vi "test_abs_mixing.vi"() -> ()   [LabVIEW 2017]
doc: "Minimal example that demonstrates functions implemented in the SorpPropLib for absorption working pairs based on the mixing approach."
panel:
  out "Mole fraction of second component":cluster{dbl[], dbl[]}[](graph)=[{[1000.0, 1001.0, 1002.0, 1003.0, 1004.0, 1005.0, 1006.0, 1007.0, 1008.0, 1009.0], [7.283559365756087e-05, 7.276280999979345e-05, 7.26901716201489e-05, 7.261767808386388e-05, 7.254532895861754e-05, 7.247312381253312e-05, 7.24010622172866e-05, 7.232914374399879e-05, 7.225736796756532e-05, 7.218573446365895e-05]}]
  out "Mole fraction of first component":cluster{dbl[], dbl[]}[](graph)=[{[1000.0, 1001.0, 1002.0, 1003.0, 1004.0, 1005.0, 1006.0, 1007.0, 1008.0, 1009.0], [0.9999271644063424, 0.9999272371900002, 0.9999273098283799, 0.9999273823219161, 0.9999274546710414, 0.9999275268761875, 0.9999275989377827, 0.999927670856256, 0.9999277426320324, 0.9999278142655363]}]
  out "Der. of pressure wrt. liquid mole fraction":cluster{dbl[], dbl[]}[](graph)=[{[1000.0, 1001.0, 1002.0, 1003.0, 1004.0, 1005.0, 1006.0, 1007.0, 1008.0, 1009.0], [401367.58805715543, 401367.0721974449, 401385.10792075976, 401372.6104574289, 401380.4616818106, 401371.28151513933, 401381.7575241774, 401382.0286104419, 401375.35766007204, 401370.0730695291]}]
  out "Der. of pressure wrt. temperature":cluster{dbl[], dbl[]}[](graph)=[{[1000.0, 1001.0, 1002.0, 1003.0, 1004.0, 1005.0, 1006.0, 1007.0, 1008.0, 1009.0], [25.245659760457784, 25.27229398367581, 25.296958770582023, 25.321660064605567, 25.347597220388707, 25.374199005341325, 25.39747936339154, 25.424986820326012, 25.4496207963939, 25.4734746010854]}]
  out "Temperature":cluster{dbl[], dbl[]}[](graph)=[{[1000.0, 1001.0, 1002.0, 1003.0, 1004.0, 1005.0, 1006.0, 1007.0, 1008.0, 1009.0], [nan, nan, nan, nan, nan, nan, nan, nan, nan, nan]}]
  out "Pressure":cluster{dbl[], dbl[]}[](graph)=[{[1000.0, 1001.0, 1002.0, 1003.0, 1004.0, 1005.0, 1006.0, 1007.0, 1008.0, 1009.0], [999.9996844004786, 1000.9996848022826, 1001.9996851320313, 1002.9996861115469, 1003.9996864578828, 1004.9996867189573, 1005.9996873328884, 1006.9996881341087, 1007.9996883623128, 1008.9996887136538]}]
  out "Liquid mole fraction":cluster{dbl[], dbl[]}[](graph)=[{[1000.0, 1001.0, 1002.0, 1003.0, 1004.0, 1005.0, 1006.0, 1007.0, 1008.0, 1009.0], [0.0024860925016939863, 0.0024885839313615603, 0.0024910753610397503, 0.002493566790576794, 0.0024960582188671056, 0.002498549646644934, 0.0025010410748412923, 0.0025035325023132905, 0.002506023929378515, 0.002508515355425353]}]
  in  "WorkingPair (Input)":T1={"no_iso"=1, "no_p_sat"=1, "path_db"="D:\\Driesel\\SorpLibLocal\\labview_wrapper\\data\\json\\sorpproplib.json", "wp_as"="lubricant", "wp_st"="POE ISO7", "wp_iso"="MixingRule", "wp_rf"="Isobutane", "rf_rhol"="NoSaturatedLiquidDensity", "no_rhol"=1, "rf_psat"="NoVaporPressure"}
  in  "Temperature in K (Input)":dbl=300.0
  in  "Pressure in Pa (Input)":dbl=1000.0
  # "Calculating temperature depending on pressure\nand molar fraction often does not converge.\n\n=> Should not be used!"
  # "Increase pressure by 10 Pa in steps of 1 Pa."
  # "Path to database"
  # "Name of sorbent"
  # "Name of sub-type of sorbent"
  # "Name of refrigerant"
  # "Name of isotherm"
  # "ID of isotherm"
  # "Name of calculation approach for vapor pressure"
  # "ID of vapor pressure equation"
  # "Name of calculation approach for liquid density"
  # "ID of liquid density equation"
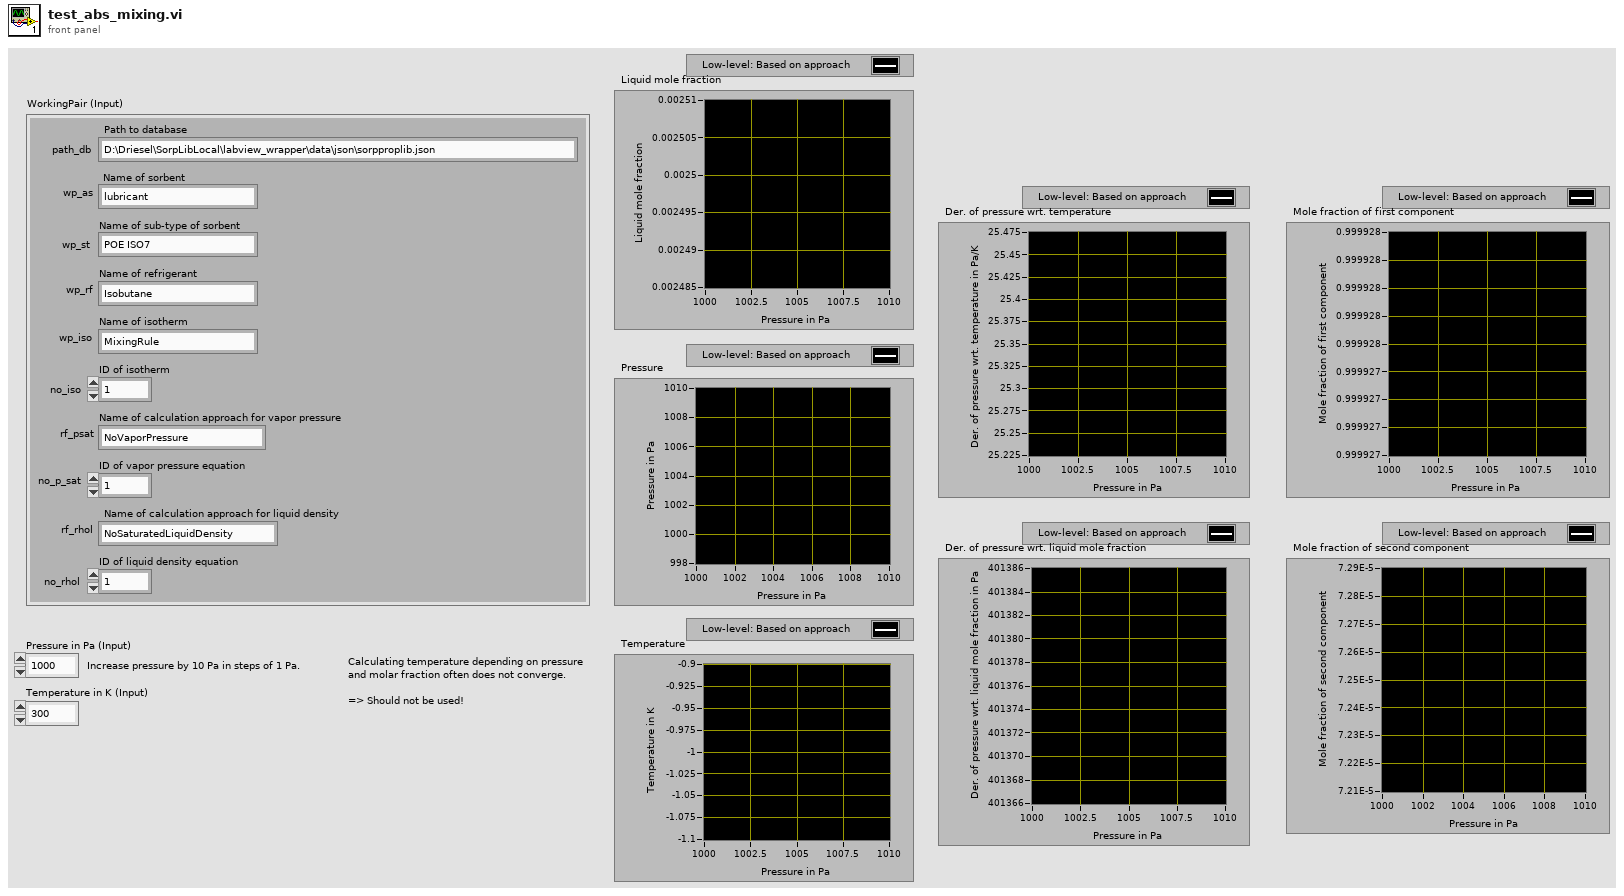
[diagram p1: front panel]
types:
  T1 = cluster{"no_iso":i32, "no_p_sat":i32, "path_db":string, "wp_as":string, "wp_st":string, "wp_iso":string, "wp_rf":string, "rf_rhol":string, "no_rhol":i32, "rf_psat":string}
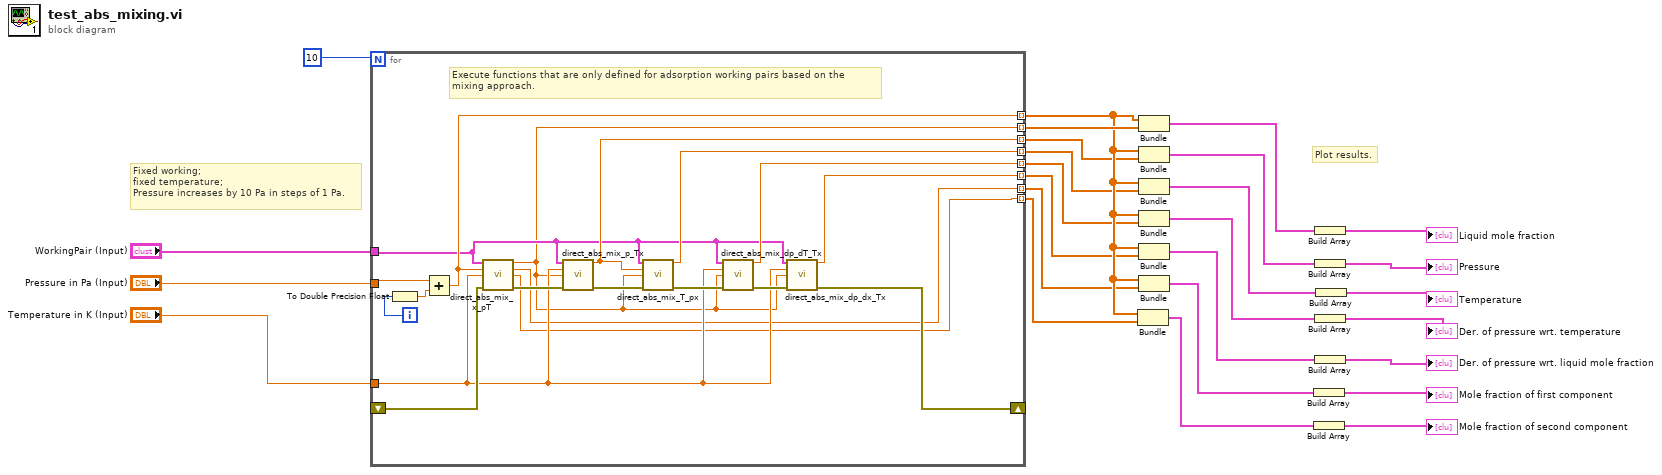
[diagram p0: block diagram]
diagram:
  # "Plot results."
  # "Fixed working;\nfixed temperature;\nPressure increases by 10 Pa in steps of 1 Pa."
  n1 = for {
    N: 10 -> [_]
    tunnel: "Pressure in Pa (Input)" -> [w45]
    tunnel: "Temperature in K (Input)" -> [w32]
    tunnel: "WorkingPair (Input)" -> [w33]
    shift-right: [w29] -> _
    shift-left: _ -> [w42]
    tunnel: [w37] -> w21 mode=indexing
    tunnel: [w41] -> w23 mode=indexing
    tunnel: [w31] -> w24 mode=indexing
    tunnel: [w39] -> w22 mode=indexing
    tunnel: [w35] -> w20 mode=indexing
    tunnel: [w30] -> w19 mode=indexing
    tunnel: [w28] -> w17 mode=indexing
    tunnel: [w27] -> w18 mode=indexing
    i -> [w44]
    # "Execute functions that are only defined for adsorption working pairs based on the\nmixing approach."
    n2 = To Double Precision Float(number=w44) -> (double precision float=w43:dbl)
    n3 = Add(x=w45, y=w43) -> (x+y=w41:dbl)
    n4 = call "direct_abs_mix_x_pT.vi"("WorkingPair (Input)"=w33, "Pressure in Pa (Input)"=w41, "Temperature in K (Input)"=w32, "Error (Input)"=w42) -> ("Mole fraction of first component liquid phase in mol/mol (Output)"=w31:dbl, "Mole fraction of first component (Output)"=w28:dbl, "Mole fraction of second component (Output)"=w27:dbl, "Error (Output)"=w40:errorcluster)  [unwired: 8 in]
    n5 = call "direct_abs_mix_p_Tx.vi"("WorkingPair (Input)"=w33, "Temperature in K (Input)"=w32, "Mole fraction in liquid phase in mol/mol (Input)"=w31, "Error (Input)"=w40) -> ("Pressure in Pa (Output)"=w39:dbl, "Error (Output)"=w38:errorcluster)  [unwired: 8 in, 2 out]
    n6 = call "direct_abs_mix_T_px.vi"("WorkingPair (Input)"=w33, "Pressure in Pa (Input)"=w39, "Mole fraction in liquid phase in mol/mol (Input)"=w31, "Error (Input)"=w38) -> ("Temperature in K (Output)"=w37:dbl, "Error (Output)"=w36:errorcluster)  [unwired: 8 in, 2 out]
    n7 = call "direct_abs_mix_dp_dT_Tx.vi"("WorkingPair (Input)"=w33, "Temperature in K (Input)"=w32, "Mole fraction in liquid phase in mol/mol (Input)"=w31, "Error (Input)"=w36) -> ("Der. of equilibrium pressure wrt temperature in Pa/K (Output)"=w35:dbl, "Error (Output)"=w34:errorcluster)  [unwired: 10 in]
    n8 = call "direct_abs_mix_dp_dx_Tx.vi"("WorkingPair (Input)"=w33, "Temperature in K (Input)"=w32, "Mole fraction in liquid phase in mol/mol (Input)"=w31, "Error (Input)"=w34) -> ("Der. of equilibrium pressure wrt liquid mole fraction in Pa (Output)"=w30:dbl, "Error (Output)"=w29:errorcluster)  [unwired: 10 in]
  }
  n9 = Bundle(w23, w18) -> (w5:cluster{dbl[], dbl[]})  [unwired: 1 in]
  n10 = Bundle(w23, w24) -> (w16:cluster{dbl[], dbl[]})  [unwired: 1 in]
  n11 = Bundle(w23, w22) -> (w15:cluster{dbl[], dbl[]})  [unwired: 1 in]
  n12 = Bundle(w23, w21) -> (w14:cluster{dbl[], dbl[]})  [unwired: 1 in]
  n13 = Bundle(w23, w20) -> (w13:cluster{dbl[], dbl[]})  [unwired: 1 in]
  n14 = Bundle(w23, w19) -> (w8:cluster{dbl[], dbl[]})  [unwired: 1 in]
  n15 = Bundle(w23, w17) -> (w6:cluster{dbl[], dbl[]})  [unwired: 1 in]
  n16 = Build Array(w6) -> (→"Mole fraction of first component":cluster{dbl[], dbl[]}[])
  n17 = Build Array(w5) -> (→"Mole fraction of second component":cluster{dbl[], dbl[]}[])
  n18 = Build Array(w16) -> (→"Liquid mole fraction":cluster{dbl[], dbl[]}[])
  n19 = Build Array(w15) -> (→"Pressure":cluster{dbl[], dbl[]}[])
  n20 = Build Array(w13) -> (→"Der. of pressure wrt. temperature":cluster{dbl[], dbl[]}[])
  n21 = Build Array(w8) -> (→"Der. of pressure wrt. liquid mole fraction":cluster{dbl[], dbl[]}[])
  n22 = Build Array(w14) -> (→"Temperature":cluster{dbl[], dbl[]}[])
